vi "Insert into subpanel.vi"(7 "Subpanel to insert into":refnum<vi>, 8 "error in (no error)":errorcluster, 10 "Clone name (blank = not cloneable)":string, 11 "Fiber Auto Collimation panel in":refnum<class "Fiber Auto Collimation panel.lvclass">) -> (0 "error out":errorcluster, 3 "Fiber Auto Collimation panel out":refnum<class "Fiber Auto Collimation panel.lvclass">)   [LabVIEW 2018, in "Fiber Auto Collimation panel.lvclass"]
doc: "Finds the running panel input passed in inside the panel run registry, and if found, attempts to insert it in the subpanel that was passed in as a reference."
uses:
  Fiber Auto Collimation panel.lvclass
  Fiber Auto Collimation panel.lvclass/Fiber Auto Collimation panel.ctl
  <vilib>/Utility/LVClass/Get LV Class Name.vi
  <vilib>/Utility/error.llb/Trim Whitespace.vi
  <userlib>/nLight Error Handling/Merge errors no loss.vi
  References/Fiber Auto Collimation References.lvclass
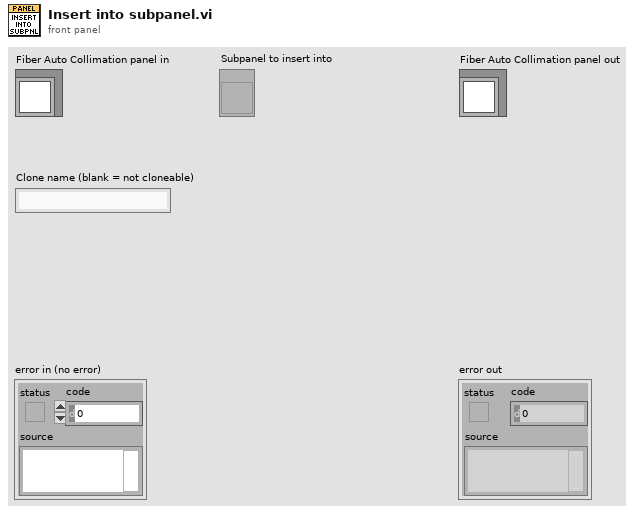
[diagram p1: front panel]
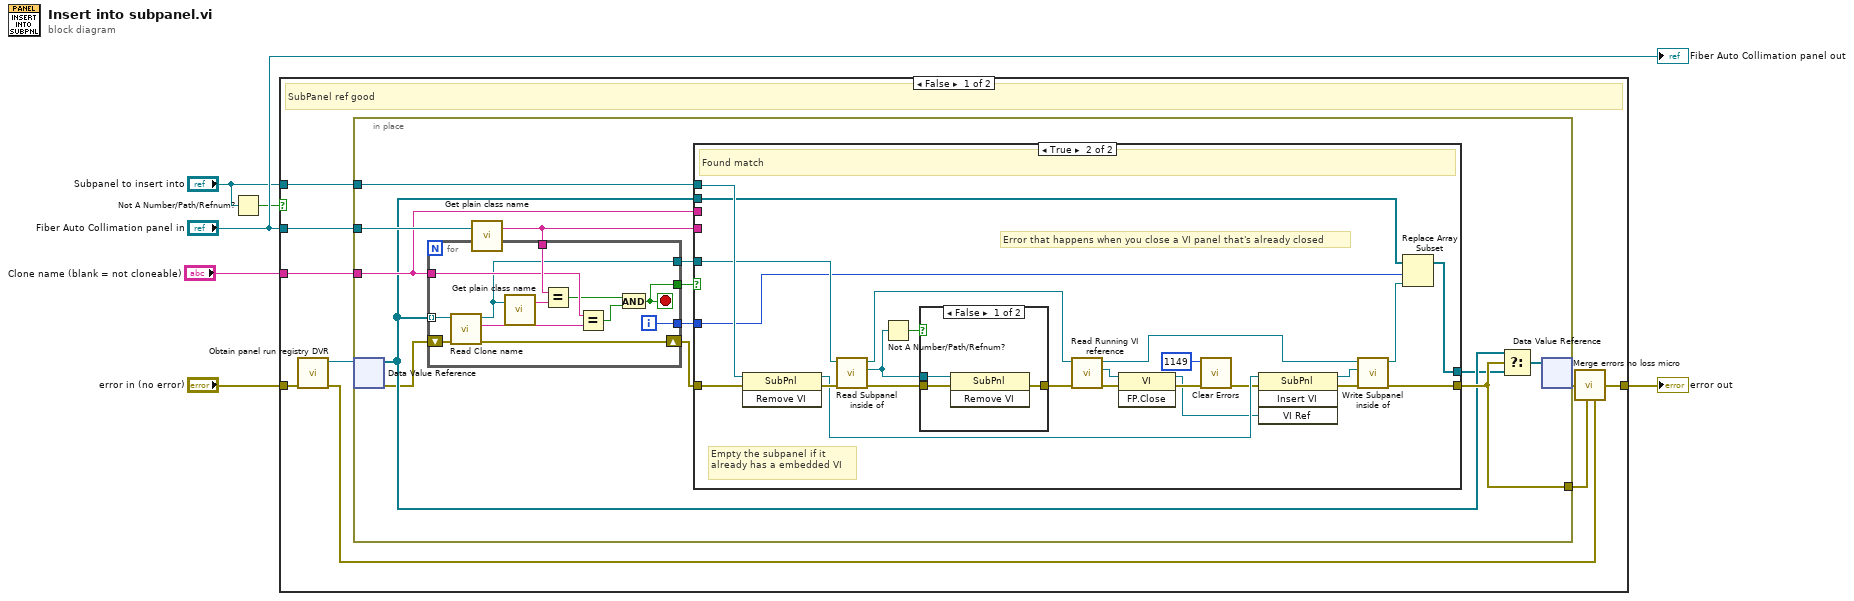
[diagram p0: block diagram]
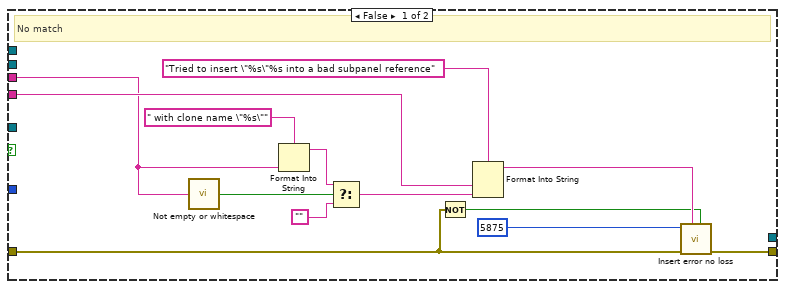
[diagram p2: hidden frame]
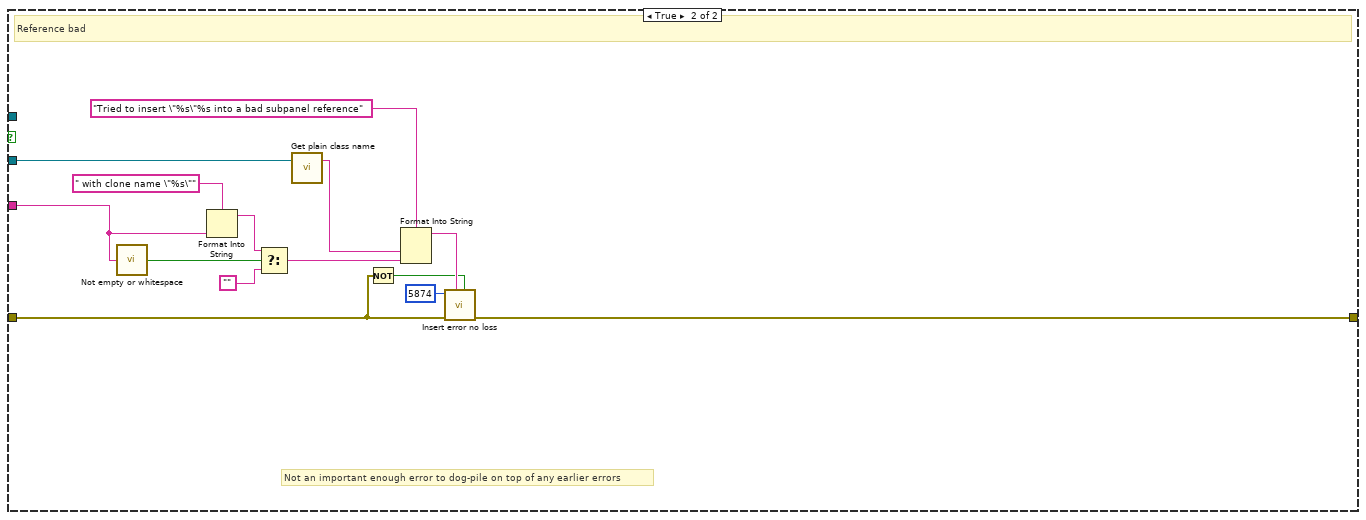
[diagram p4: hidden frame]
diagram:
  n1 = Not A Number/Path/Refnum?(number/path/refnum="Subpanel to insert into") -> (NaN/Path/Refnum?=w2:bool)
  n2 = case shown="False" w2 {
    tunnel: "error in (no error)" -> [w14 w84]
    tunnel: "Clone name (blank = not cloneable)" -> [w13 w89]
    tunnel: "Fiber Auto Collimation panel in" -> [w12 w94]
    tunnel: "Subpanel to insert into" -> [w11 _]
    tunnel: [w7 w82] -> w1
    frame False {
      # "SubPanel ref good"
      n3 = call "Obtain panel run registry DVR.vi"("error in"=w14) -> ("error out"=w9:errorcluster, "Panel registration DVR"=w15:refnum<data-value>)  [unwired: 9 in]
      n4 = in-place {
        in-place-border: [w22] -> w10
        in-place-border: w12 -> [w28]
        in-place-border: w13 -> [w25]
        in-place-border: w11 -> [w23]
        n5 = in-place-dvr #1(w15) -> (w21:refnum<class "Fiber Auto Collimation panel.lvclass">[], w17:errorcluster)
        n6 = call <userlib>:"Get plain class name.vi"("Any class"=w28) -> ("Plain class name"=w26:string)  [unwired: 2 in]
        n7 = for {
          tunnel: w21 -> [w81] mode=indexing
          tunnel: w26 -> [w79]
          tunnel: w25 -> [w77]
          tunnel: [w74] -> w27
          tunnel: [w73] -> w19
          tunnel: [w72] -> w24
          shift-right: [w70] -> w16
          shift-left: w17 -> [w71]
          i -> [w73]
          stop <- w74 stop-if-true
          n8 = call "Read Clone name.vi"("error in (no error)"=w71, "Fiber Auto Collimation panel in"=w81) -> ("error out"=w70:errorcluster, "Clone name"=w78:string, "Fiber Auto Collimation panel out"=w72:refnum<class "Fiber Auto Collimation panel.lvclass">)  [unwired: 7 in]
          n9 = call <userlib>:"Get plain class name.vi"("Any class"=w72) -> ("Plain class name"=w80:string)  [unwired: 2 in]
          n10 = Equal?(x=w79, y=w80) -> (x = y?=w75:bool)
          n11 = Equal?(x=w77, y=w78) -> (x = y?=w76:bool)
          n12 = And(x=w75, y=w76) -> (x .and. y?=w74:bool)
        }
        n13 = case shown="True" w27 {
          tunnel: w16 -> [w32 w64]
          tunnel: [w31 w49] -> w22
          tunnel: w26 -> [w30 _]
          tunnel: w25 -> [w29 _]
          tunnel: w24 -> [_ w62]
          tunnel: w23 -> [_ w65]
          tunnel: w21 -> [_ w48]
          tunnel: w19 -> [_ w47]
          tunnel: [_ w45] -> w18
          frame False {
            # "No match"
            n14 = call <userlib>:"Not empty or whitespace.vi"("String"=w29) -> ("Not empty or all whitespace"=w39:bool)  [unwired: 4 in]
            n15 = Format Into String(format string=" with clone name \"%s\"", w29) -> (resulting string=w37:string)  [unwired: 2 in, 1 out]
            n16 = Select(t=w37, s=w39, f="") -> (s? t:f=w35:string)
            n17 = Not(x=w32) -> (.not. x?=w33:bool)
            n18 = Format Into String(format string="Tried to insert \"%s\"%s into a bad subpanel reference", w30, w35) -> (resulting string=w34:string)  [unwired: 2 in, 1 out]
            n19 = call <userlib>:"Insert error no loss.vi"("Add error? (T)"=w33, "error message"=w34, "error in (no error)"=w32, "error code"=5875) -> ("error out"=w31:errorcluster)  [unwired: 5 in]
          }
          frame True {
            # "Error that happens when you close a VI panel that's already closed"
            # "Empty the subpanel if it already has a embedded VI"
            # "Found match"
            n20 = invoke class="SubPnl" method="Remove VI"(reference=w65, error in=w64) -> (reference out=w53:refnum<vi>, error out=w63:errorcluster)  [unwired: 1 in, 1 out]
            n21 = call "Read Subpanel inside of.vi"("error in (no error)"=w63, "Fiber Auto Collimation panel in"=w62) -> ("error out"=w60:errorcluster, "Subpanel inside of"=w59:refnum<vi>, "Fiber Auto Collimation panel out"=w57:refnum<class "Fiber Auto Collimation panel.lvclass">)  [unwired: 7 in]
            n22 = Not A Number/Path/Refnum?(number/path/refnum=w59) -> (NaN/Path/Refnum?=w61:bool)
            n23 = case shown="False" w61 {
              tunnel: w60 -> [w68 w69]
              tunnel: w59 -> [w67 _]
              tunnel: [w66 w69] -> w58
              frame False {
                n24 = invoke class="SubPnl" method="Remove VI"(reference=w67, error in=w68) -> (error out=w66:errorcluster)  [unwired: 1 in, 2 out]
              }
              frame True {
              }
            }
            n25 = call "Read Running VI reference.vi"("error in (no error)"=w58, "Fiber Auto Collimation panel in"=w57) -> ("error out"=w56:errorcluster, "Running VI reference"=w55:refnum<vi>, "Fiber Auto Collimation panel out"=w44:refnum<class "Fiber Auto Collimation panel.lvclass">)  [unwired: 7 in]
            n26 = invoke class="VI" method="FP.Close"(reference=w55, error in=w56) -> (reference out=w52:refnum<vi>, error out=w54:errorcluster)  [unwired: 1 in, 1 out]
            n27 = call <vilib>:"Clear Errors.vi"("error in (no error)"=w54, "specific error code to clear (0: all)"=1149) -> ("error out"=w43:errorcluster)  [unwired: 4 in, 1 out]
            n28 = invoke class="SubPnl" method="Insert VI"(reference=w53, error in=w43, "VI Ref"=w52) -> (reference out=w50:refnum<vi>, error out=w51:errorcluster)  [unwired: 1 in, 2 out]
            n29 = call "Write Subpanel inside of.vi"("error in (no error)"=w51, "Subpanel inside of"=w50, "Fiber Auto Collimation panel in"=w44) -> ("error out"=w49:errorcluster, "Fiber Auto Collimation panel out"=w46:refnum<class "Fiber Auto Collimation panel.lvclass">)  [unwired: 7 in]
            n30 = Replace Array Subset(array=w48, new element=w46, index=w47) -> (w45:refnum<class "Fiber Auto Collimation panel.lvclass">[])
          }
        }
        n31 = Select(t=w21, s=w22, f=w18) -> (s? t:f=w20:refnum<class "Fiber Auto Collimation panel.lvclass">[])
        n32 = in-place-dvr #1(w20) -> (w8:errorcluster)  [unwired: 1 out]
      }
      n33 = call <userlib>:"Merge errors no loss micro.vi"("error in (no error) 1"=w8, "error in (no error) 5"=w10, "error in (no error) 6"=w9) -> ("error out"=w7:errorcluster)  [unwired: 6 in]
    }
    frame True {
      # "Not an important enough error to dog-pile on top of any earlier errors"
      # "Reference bad"
      n34 = call <userlib>:"Not empty or whitespace.vi"("String"=w89) -> ("Not empty or all whitespace"=w92:bool)  [unwired: 4 in]
      n35 = Format Into String(format string=" with clone name \"%s\"", w89) -> (resulting string=w90:string)  [unwired: 2 in, 1 out]
      n36 = Select(t=w90, s=w92, f="") -> (s? t:f=w87:string)
      n37 = call <userlib>:"Get plain class name.vi"("Any class"=w94) -> ("Plain class name"=w86:string)  [unwired: 2 in]
      n38 = Not(x=w84) -> (.not. x?=w83:bool)
      n39 = Format Into String(format string="Tried to insert \"%s\"%s into a bad subpanel reference", w86, w87) -> (resulting string=w85:string)  [unwired: 2 in, 1 out]
      n40 = call <userlib>:"Insert error no loss.vi"("Add error? (T)"=w83, "error message"=w85, "error in (no error)"=w84, "error code"=5874) -> ("error out"=w82:errorcluster)  [unwired: 5 in]
    }
  }
  "error out" <- w1
  "Fiber Auto Collimation panel out" <- "Fiber Auto Collimation panel in"
